vi "Render.vi"(7 "Renderer":refnum<class "Renderer.lvclass">, 8 "error in (no error)":errorcluster, 10 "Camera":refnum<class "Camera.lvclass">, 11 "Ship in":refnum<class "Ship.lvclass">) -> (0 "error out":errorcluster)   [LabVIEW 2021, in "Ship.lvclass"]
uses:
  Ship.lvclass
  Camera/Camera.lvclass
  Renderer/Renderer.lvclass
  Ship.lvclass/Ship.ctl
  LabSDL2/Source/Libraries/LibSDL2 Wrapper/LibSDL2.lvlib
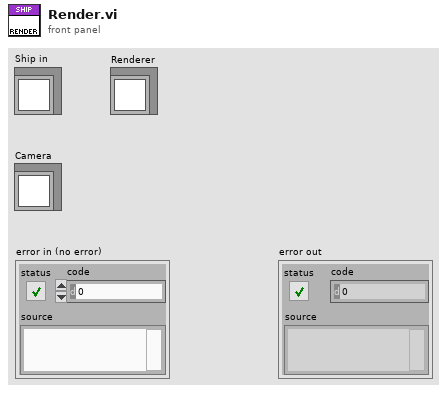
[diagram p1: front panel]
types:
  T1 = typedef "LibSDL2.lvlib/Rectangle.ctl" = cluster{"x":i32, "y":i32, "Width":i32, "Height":i32}
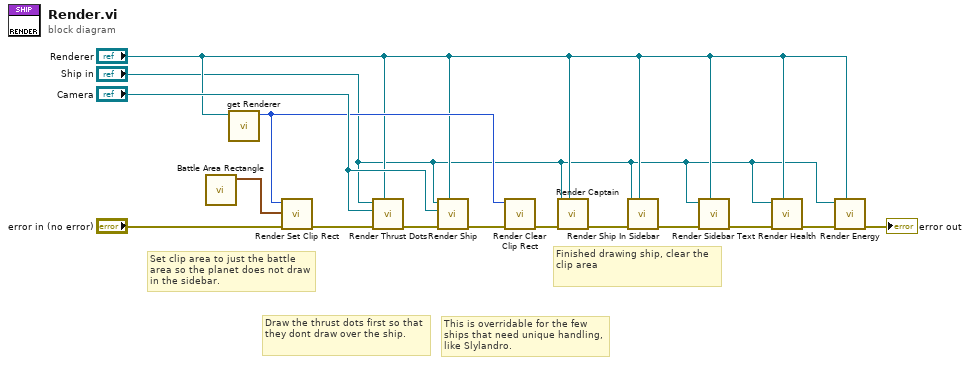
[diagram p0: block diagram]
diagram:
  # "This is overridable for the few ships that need unique handling, like Slylandro."
  # "Finished drawing ship, clear the clip area"
  # "Set clip area to just the battle area so the planet does not draw in the sidebar."
  # "Draw the thrust dots first so that they dont draw over the ship."
  n1 = call "Battle Area Rectangle.vi"() -> ("Viewport"=w6:T1)  [unwired: 11 in]
  n2 = call-dynamic "get Renderer.vi"("Renderer in"="Renderer") -> ("Renderer"=w7:u32)  [unwired: 10 in]
  n3 = call "Render Set Clip Rect.vi"("error in"="error in (no error)", "Rectangle"=w6, "Renderer Pointer"=w7) -> ("error out"=w13:errorcluster)  [unwired: 7 in, 1 out]
  n4 = call "Render Thrust Dots.vi"("Renderer"="Renderer", "error in (no error)"=w13, "Camera"="Camera", "Ship in"="Ship in") -> ("error out"=w14:errorcluster)  [unwired: 7 in]
  n5 = call-dynamic "Render Ship.vi"("Renderer"="Renderer", "error in (no error)"=w14, "Camera"="Camera", "Ship in"="Ship in") -> ("error out"=w10:errorcluster)  [unwired: 7 in]
  n6 = call "Render Clear Clip Rect.vi"("error in"=w10, "Renderer Pointer"=w7) -> ("error out"=w9:errorcluster)  [unwired: 8 in, 1 out]
  n7 = call "Render Captain.vi"("Renderer"="Renderer", "error in (no error)"=w9, "Ship in"="Ship in") -> ("error out"=w12:errorcluster)  [unwired: 8 in]
  n8 = call "Render Ship In Sidebar.vi"("Renderer"="Renderer", "error in (no error)"=w12, "Ship in"="Ship in") -> ("error out"=w11:errorcluster)  [unwired: 8 in]
  n9 = call "Render Sidebar Text.vi"("Renderer"="Renderer", "error in (no error)"=w11, "Ship in"="Ship in") -> ("error out"=w5:errorcluster)  [unwired: 8 in]
  n10 = call "Render Health.vi"("Renderer"="Renderer", "error in (no error)"=w5, "Ship in"="Ship in") -> ("error out"=w4:errorcluster)  [unwired: 8 in]
  n11 = call "Render Energy.vi"("Renderer"="Renderer", "error in (no error)"=w4, "Ship in"="Ship in") -> ("error out"=→"error out":errorcluster)  [unwired: 8 in]
